vi "Filter Dev Nodes.vi"(10 "All Dev Nodes":T1[](array[typedef]) {"Force Bridge"."scaling information"."physical units" items=["Newtons"=15875, "Pounds"=15876, "kgf"=15877]; "Force Bridge"."scaling information"."electrical units" items=["Volts/Volt"=15896, "mVolts/Volt"=15897]; "Force Bridge"."bridge information"."voltage excitation source" items=["Internal"=10200, "External"=10167]; "Force Bridge"."bridge information"."bridge configuration" items=["Full Bridge"=10182, "Half Bridge"=10187, "Quarter Bridge"=10270]; "Conversion"."ScaleOffset" format="%.3f"; "Conversion"."MinEngUnit" format="%.3f"; "Conversion"."MaxEngUnit" format="%.3f"; "Conversion"."MinSignal" format="%.3f"; "Conversion"."MaxSignal" format="%.3f"; "Terminal Configuration" items=["default"=-1, "RSE"=10083, "NRSE"=10078, "Differential"=10106, "Pseudodifferential"=12529]}, 11 "DevName":string) -> (2 "Filtered Dev Nodes":T1[](array[typedef]) {"Force Bridge"."scaling information"."physical units" items=["Newtons"=15875, "Pounds"=15876, "kgf"=15877]; "Force Bridge"."scaling information"."electrical units" items=["Volts/Volt"=15896, "mVolts/Volt"=15897]; "Force Bridge"."bridge information"."voltage excitation source" items=["Internal"=10200, "External"=10167]; "Force Bridge"."bridge information"."bridge configuration" items=["Full Bridge"=10182, "Half Bridge"=10187, "Quarter Bridge"=10270]; "Conversion"."ScaleOffset" format="%.3f"; "Conversion"."MinEngUnit" format="%.3f"; "Conversion"."MaxEngUnit" format="%.3f"; "Conversion"."MinSignal" format="%.3f"; "Conversion"."MaxSignal" format="%.3f"; "Terminal Configuration" items=["default"=-1, "RSE"=10083, "NRSE"=10078, "Differential"=10106, "Pseudodifferential"=12529]}, 3 "DevName out":string)   [LabVIEW 2017, in "DAQ.lvclass"]
doc: "Developed by Kevin Thompson\nkevin@thompsonengineering.net\n\nCopyright 2018-2020\nThompson Engineering, LLC"
uses:
  DAQ.lvclass
  DataTypes/TD AI Channel--cluster.ctl
  DataTypes/TD DataValueConversion--cluster.ctl
  DataTypes/TD AI DAQ Type--enum.ctl
  DataTypes/TD AI Force Bridge--cluster.ctl
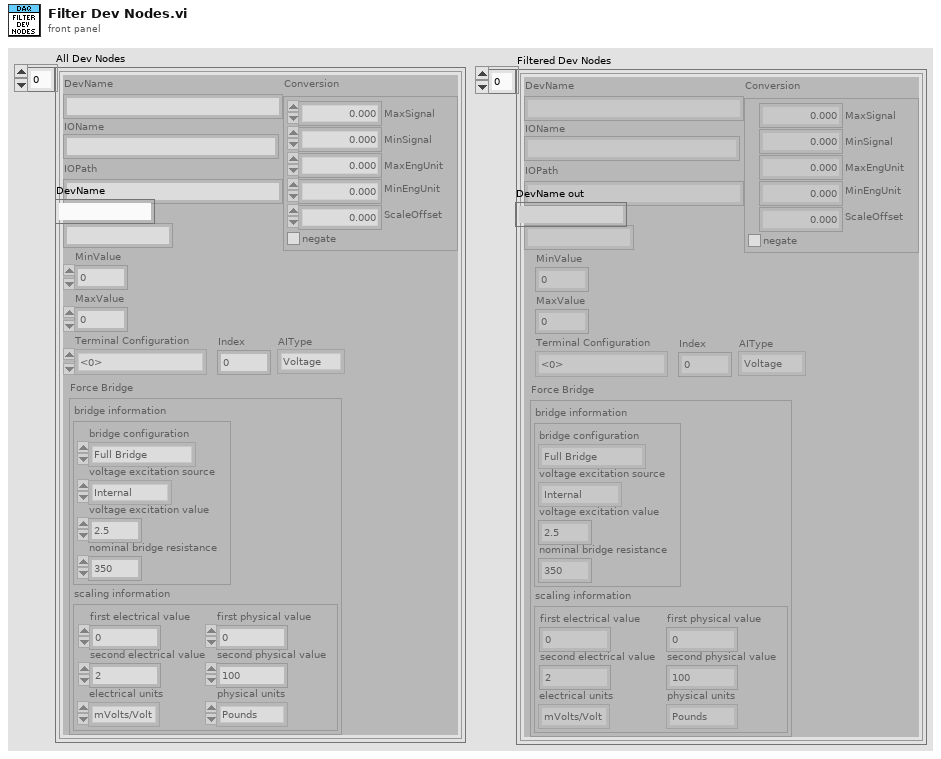
[diagram p1: front panel]
types:
  T1 = typedef "DAQ.lvclass/TD AI Channel--cluster.ctl" = cluster{"DevName":string, "IOName":string, "IOPath":string, "SchemName":string, "MinValue":dbl, "MaxValue":dbl, "Terminal Configuration":i32, "Index":i32, "Conversion":T2, "AIType":T3, "Force Bridge":T4}
  T2 = typedef "DAQ.lvclass/TD DataValueConversion--cluster.ctl" = cluster{"MaxSignal":dbl, "MinSignal":dbl, "MaxEngUnit":dbl, "MinEngUnit":dbl, "ScaleOffset":dbl, "negate":bool}
  T3 = typedef "DAQ.lvclass/TD AI DAQ Type--enum.ctl" = enum16{"Voltage", "Current", "Strain Gage", "Force Bridge"}
  T4 = typedef "DAQ.lvclass/TD AI Force Bridge--cluster.ctl" = cluster{"bridge information":cluster{"bridge configuration":i32, "voltage excitation source":i32, "voltage excitation value":dbl, "nominal bridge resistance":dbl}, "scaling information":cluster{"first electrical value":dbl, "second electrical value":dbl, "electrical units":i32, "first physical value":dbl, "second physical value":dbl, "physical units":i32}}
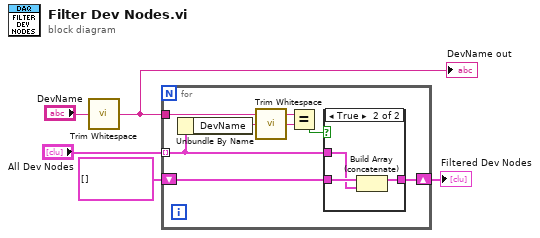
[diagram p0: block diagram]
diagram:
  n1 = call <vilib>:"Trim Whitespace.vi"("string"="DevName") -> ("trimmed string"=w3:string)  [unwired: 1 in]
  "DevName out" <- w3
  n2 = for {
    tunnel: "All Dev Nodes" -> [w11] mode=indexing
    shift-right: [w9] -> w1
    shift-left: T1[] [] ("Dev Nodes") -> [w10]
    tunnel: w3 -> [w7]
    n3 = Unbundle By Name(w11) -> ("DevName"=w12:string)
    n4 = call <vilib>:"Trim Whitespace.vi"("string"=w12) -> ("trimmed string"=w8:string)  [unwired: 1 in]
    n5 = Equal?(x=w7, y=w8) -> (x = y?=w6:bool)
    n6 = case shown="True" w6 {
      tunnel: w11 -> [_ w14]
      tunnel: w10 -> [w13 w16]
      tunnel: [w13 w15] -> w9
      frame False {
      }
      frame True {
        n7 = Build Array (concatenate)(w16, w14) -> (w15:T1[])
      }
    }
  }
  "Filtered Dev Nodes" <- w1
